vi "state_index.vi"(11 "4 x U32 2":u32[](array[numeric]) format="%.0x") -> (3 "j":u64)   [LabVIEW 2017]
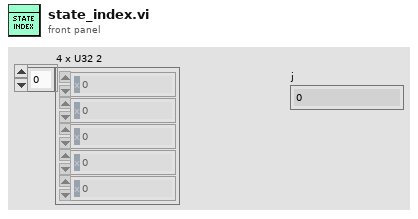
[diagram p1: front panel]
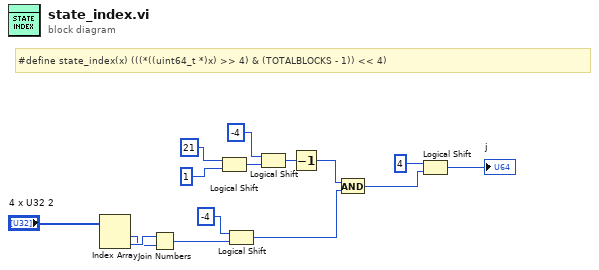
[diagram p0: block diagram]
diagram:
  # "#define state_index(x) (((*((uint64_t *)x) >> 4) & (TOTALBLOCKS - 1)) << 4)"
  n1 = Index Array(array="4 x U32 2") -> (element #1=w3:u32, element #2=w4:u32)  [unwired: 2 in]
  n2 = Join Numbers(hi=w4, lo=w3) -> ((hi.lo)=w2:u64)
  n3 = Logical Shift(y=i16 21, x=1) -> (x << y=w12:i32)
  n4 = Logical Shift(y=i16 -4, x=w2) -> (x << y=w5:u64)
  n5 = Logical Shift(y=i16 -4, x=w12) -> (x << y=w14:i32)
  n6 = Decrement(x=w14) -> (x-1=w10:i32)
  n7 = And(x=w10, y=w5) -> (x .and. y?=w11:u64)
  n8 = Logical Shift(y=i16 4, x=w11) -> (x << y=→"j":u64)
